vi "Get ToolStripProgressBar Value.vi"(8 "error in (no error)":errorcluster caption="错误输入（无错误）", 11 "ToolStripProgressBar 输入":refnum<class "ToolStripProgressBar.lvclass"> caption="DNL_LabVIEW Object in") -> (0 "error out":errorcluster caption="错误输出", 2 "Value":i32, 3 "ToolStripProgressBar 输出":refnum<class "ToolStripProgressBar.lvclass"> caption="DNL_LabVIEW Object out")   [LabVIEW 2013, in "ToolStripProgressBar.lvclass"]
uses:
  ToolStripProgressBar.lvclass
  ToolStripProgressBar.lvclass/ToolStripProgressBar.ctl
  System.Windows.Forms
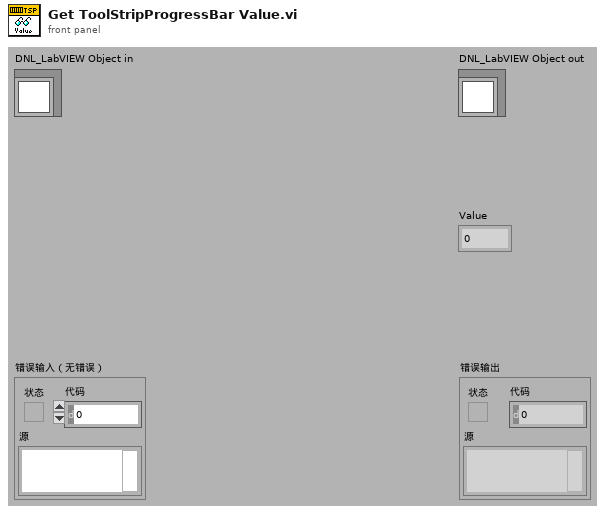
[diagram p1: front panel]
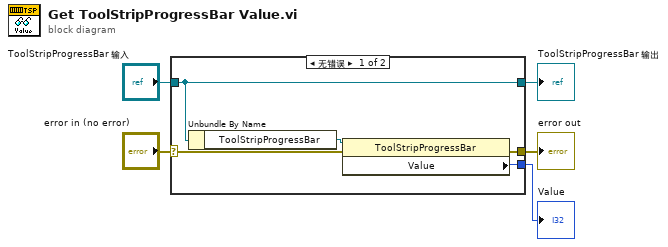
[diagram p0: block diagram]
diagram:
  n1 = case shown="无错误" "error in (no error)" {
    selector: "error in (no error)" -> [w7 w12]
    tunnel: [w6 w12] -> w4
    tunnel: [w10 w11] -> w2
    tunnel: "ToolStripProgressBar 输入" -> [w10 w11]
    tunnel: [w8 _] -> w1
    frame No Error {
      n2 = Unbundle By Name(w10) -> ("ToolStripProgressBar"=w9:refnum<k24>)
      n3 = property class="ToolStripProgressBar"(reference=w9, error in=w7) -> (error out=w6:errorcluster, "Value"=w8:i32)  [unwired: 1 out]
    }
    frame Error {
    }
  }
  "error out" <- w4
  "ToolStripProgressBar 输出" <- w2
  "Value" <- w1
